vi "InitDrive.vi"   [LabVIEW 2019]
uses:
  <vilib>/Rock Robotics/WPI/ThirdParty/REV Robotics/SPARK MAX/Typedef/Spark MAX Idle Mode.ctl
  refnums.vi
types:
  T1 = typedef "Spark MAX Idle Mode.ctl" = enum16{"Coast", "Brake"}
  T2 = typedef "WPI_MotorControlDeviceRef.ctl" = cluster{"DeviceStatus":errorcluster, "Type":T3, "PWM":cluster{"PWM Channel":T4, "DeadBand":T5}, "CAN":cluster{"Device Number":u8, "SetOutput VI Ref":variant, "GetOutput VI Ref":variant, "Enable VI Ref":variant, "Disable VI Ref":variant, "Data":variant}, "Invert":bool, "DIO PWM":cluster{"PWM \"Enable\" Channel":T4, "DIOChannel":T6, "PWM Rate":dbl}}
  T3 = typedef "WPI_MotorControlType.ctl" = enum16{"PWM", "CAN", "DIO PWM"}
  T4 = typedef "FPGA_DIOPWMChannel.ctl" = enum8{"PWM 0", "PWM 1", "PWM 2", "PWM 3", "PWM 4", "PWM 5", "PWM 6", "PWM 7", "PWM 8", "PWM 9", "PWM MXP 0", "PWM MXP 1", "PWM MXP 2", "PWM MXP 3", "PWM MXP 4", "PWM MXP 5", "PWM MXP 6", "PWM MXP 7", "PWM MXP 8", "PWM MXP 9", "Invalid"}
  T5 = typedef "WPI_PWMDeadband.ctl" = cluster{"Name":string, "maxPositivePwm":i32, "minPositivePwm":i32, "centerPwm":i32, "maxNegativePwm":i32, "minNegativePwm":i32, "angularRange":u16}
  T6 = typedef "FPGA_DIOChannel.ctl" = enum8{"DIO 0", "DIO 1", "DIO 2", "DIO 3", "DIO 4", "DIO 5", "DIO 6", "DIO 7", "DIO 8", "DIO 9", "DIO MXP 0", "DIO MXP 1", "DIO MXP 2", "DIO MXP 3", "DIO MXP 4", "DIO MXP 5", "DIO MXP 6", "DIO MXP 7", "DIO MXP 8", "DIO MXP 9", "DIO MXP 10", "DIO MXP 11", "DIO MXP 12", "DIO MXP 13", "DIO MXP 14", "DIO MXP 15", "SPI Port CS1", "SPI Port CS2", "SPI Port CS3", "SPI Port MISO", "SPI Port MOSI", "Invalid"}
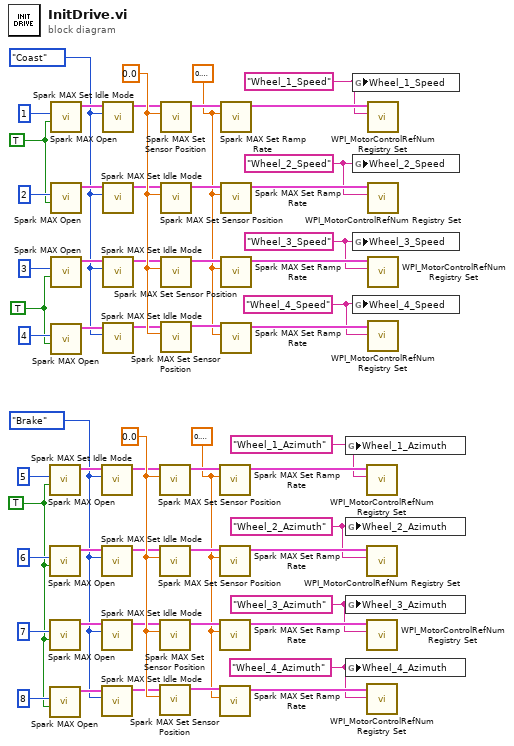
[diagram p0: block diagram]
diagram:
  w1 = TRUE
  w29 = 0.0
  w3 = TRUE
  w5 = "Wheel_3_Azimuth" ("refnum name")
  w4 = "Wheel_4_Azimuth" ("refnum name")
  w6 = "Wheel_2_Azimuth" ("refnum name")
  w2 = Spark_MAX_Idle_Mode."Brake" ("Idle Mode")
  w7 = "Wheel_1_Azimuth" ("refnum name")
  w8 = sgl 0.1 ("Seconds from neutral to full (0)")
  w57 = 0.0
  w31 = TRUE
  w33 = "Wheel_3_Speed" ("refnum name")
  w32 = "Wheel_4_Speed" ("refnum name")
  w34 = "Wheel_2_Speed" ("refnum name")
  w30 = Spark_MAX_Idle_Mode."Coast" ("Idle Mode")
  w35 = "Wheel_1_Speed" ("refnum name")
  w36 = sgl 0.2 ("Seconds from neutral to full (0)")
  n1 = call <vilib>:"Spark MAX Open.vi"("Invert"=w3, "Device Number"=u8 5 ("Drive 1R")) -> ("MotorControlDeviceRef"=w9:T2)  [unwired: 8 in, 1 out]
  n2 = call <vilib>:"Spark MAX Open.vi"("Invert"=w3, "Device Number"=u8 6 ("Drive 2R")) -> ("MotorControlDeviceRef"=w12:T2)  [unwired: 8 in, 1 out]
  n3 = call <vilib>:"Spark MAX Open.vi"("Invert"=w3, "Device Number"=u8 7 ("Drive  3R")) -> ("MotorControlDeviceRef"=w18:T2)  [unwired: 8 in, 1 out]
  n4 = call <vilib>:"Spark MAX Open.vi"("Invert"=w3, "Device Number"=u8 8 ("Drive 4L")) -> ("MotorControlDeviceRef"=w15:T2)  [unwired: 8 in, 1 out]
  n5 = call <vilib>:"Spark MAX Open.vi"("Invert"=w31, "Device Number"=u8 1 ("Drive 1R")) -> ("MotorControlDeviceRef"=w37:T2)  [unwired: 8 in, 1 out]
  n6 = call <vilib>:"Spark MAX Open.vi"("Invert"=w31, "Device Number"=u8 2 ("Drive 2R")) -> ("MotorControlDeviceRef"=w40:T2)  [unwired: 8 in, 1 out]
  n7 = call <vilib>:"Spark MAX Open.vi"("Invert"=w1, "Device Number"=u8 3 ("Drive  3R")) -> ("MotorControlDeviceRef"=w46:T2)  [unwired: 8 in, 1 out]
  n8 = call <vilib>:"Spark MAX Open.vi"("Invert"=w1, "Device Number"=u8 4 ("Drive 4L")) -> ("MotorControlDeviceRef"=w43:T2)  [unwired: 8 in, 1 out]
  n9 = call <vilib>:"Spark MAX Set Idle Mode.vi"("Idle Mode"=w2, "MotorControlDeviceRef in"=w9) -> ("MotorControlDeviceRef out"=w21:T2)  [unwired: 8 in, 1 out]
  n10 = call <vilib>:"Spark MAX Set Idle Mode.vi"("Idle Mode"=w2, "MotorControlDeviceRef in"=w12) -> ("MotorControlDeviceRef out"=w23:T2)  [unwired: 8 in, 1 out]
  n11 = call <vilib>:"Spark MAX Set Idle Mode.vi"("Idle Mode"=w2, "MotorControlDeviceRef in"=w18) -> ("MotorControlDeviceRef out"=w25:T2)  [unwired: 8 in, 1 out]
  n12 = call <vilib>:"Spark MAX Set Idle Mode.vi"("Idle Mode"=w2, "MotorControlDeviceRef in"=w15) -> ("MotorControlDeviceRef out"=w27:T2)  [unwired: 8 in, 1 out]
  n13 = call <vilib>:"Spark MAX Set Idle Mode.vi"("Idle Mode"=w30, "MotorControlDeviceRef in"=w37) -> ("MotorControlDeviceRef out"=w49:T2)  [unwired: 8 in, 1 out]
  n14 = call <vilib>:"Spark MAX Set Idle Mode.vi"("Idle Mode"=w30, "MotorControlDeviceRef in"=w40) -> ("MotorControlDeviceRef out"=w51:T2)  [unwired: 8 in, 1 out]
  n15 = call <vilib>:"Spark MAX Set Idle Mode.vi"("Idle Mode"=w30, "MotorControlDeviceRef in"=w46) -> ("MotorControlDeviceRef out"=w53:T2)  [unwired: 8 in, 1 out]
  n16 = call <vilib>:"Spark MAX Set Idle Mode.vi"("Idle Mode"=w30, "MotorControlDeviceRef in"=w43) -> ("MotorControlDeviceRef out"=w55:T2)  [unwired: 8 in, 1 out]
  n17 = call <vilib>:"Spark MAX Set Sensor Position.vi"("Position"=w29, "MotorControlDeviceRef"=w21) -> ("MotorControlDeviceRef"=w22:T2)  [unwired: 8 in, 1 out]
  n18 = call <vilib>:"Spark MAX Set Sensor Position.vi"("Position"=w29, "MotorControlDeviceRef"=w23) -> ("MotorControlDeviceRef"=w24:T2)  [unwired: 8 in, 1 out]
  n19 = call <vilib>:"Spark MAX Set Sensor Position.vi"("Position"=w29, "MotorControlDeviceRef"=w25) -> ("MotorControlDeviceRef"=w26:T2)  [unwired: 8 in, 1 out]
  n20 = call <vilib>:"Spark MAX Set Sensor Position.vi"("Position"=w29, "MotorControlDeviceRef"=w27) -> ("MotorControlDeviceRef"=w28:T2)  [unwired: 8 in, 1 out]
  n21 = call <vilib>:"Spark MAX Set Sensor Position.vi"("Position"=w57, "MotorControlDeviceRef"=w49) -> ("MotorControlDeviceRef"=w50:T2)  [unwired: 8 in, 1 out]
  n22 = call <vilib>:"Spark MAX Set Sensor Position.vi"("Position"=w57, "MotorControlDeviceRef"=w51) -> ("MotorControlDeviceRef"=w52:T2)  [unwired: 8 in, 1 out]
  n23 = call <vilib>:"Spark MAX Set Sensor Position.vi"("Position"=w57, "MotorControlDeviceRef"=w53) -> ("MotorControlDeviceRef"=w54:T2)  [unwired: 8 in, 1 out]
  n24 = call <vilib>:"Spark MAX Set Sensor Position.vi"("Position"=w57, "MotorControlDeviceRef"=w55) -> ("MotorControlDeviceRef"=w56:T2)  [unwired: 8 in, 1 out]
  n25 = call <vilib>:"Spark MAX Set Ramp Rate.vi"("Seconds from neutral to full (0)"=w8, "MotorControlDeviceRef in"=w22) -> ("MotorControlDeviceRef"=w10:T2)  [unwired: 8 in, 1 out]
  n26 = call <vilib>:"Spark MAX Set Ramp Rate.vi"("Seconds from neutral to full (0)"=w8, "MotorControlDeviceRef in"=w24) -> ("MotorControlDeviceRef"=w14:T2)  [unwired: 8 in, 1 out]
  n27 = call <vilib>:"Spark MAX Set Ramp Rate.vi"("Seconds from neutral to full (0)"=w8, "MotorControlDeviceRef in"=w26) -> ("MotorControlDeviceRef"=w20:T2)  [unwired: 8 in, 1 out]
  n28 = call <vilib>:"Spark MAX Set Ramp Rate.vi"("Seconds from neutral to full (0)"=w8, "MotorControlDeviceRef in"=w28) -> ("MotorControlDeviceRef"=w17:T2)  [unwired: 8 in, 1 out]
  n29 = call <vilib>:"Spark MAX Set Ramp Rate.vi"("Seconds from neutral to full (0)"=w36, "MotorControlDeviceRef in"=w50) -> ("MotorControlDeviceRef"=w38:T2)  [unwired: 8 in, 1 out]
  n30 = call <vilib>:"Spark MAX Set Ramp Rate.vi"("Seconds from neutral to full (0)"=w36, "MotorControlDeviceRef in"=w52) -> ("MotorControlDeviceRef"=w42:T2)  [unwired: 8 in, 1 out]
  n31 = call <vilib>:"Spark MAX Set Ramp Rate.vi"("Seconds from neutral to full (0)"=w36, "MotorControlDeviceRef in"=w54) -> ("MotorControlDeviceRef"=w48:T2)  [unwired: 8 in, 1 out]
  n32 = call <vilib>:"Spark MAX Set Ramp Rate.vi"("Seconds from neutral to full (0)"=w36, "MotorControlDeviceRef in"=w56) -> ("MotorControlDeviceRef"=w45:T2)  [unwired: 8 in, 1 out]
  n33 = global write "refnums.vi" "Wheel_1_Azimuth"(w7) -> ()
  n34 = global write "refnums.vi" "Wheel_2_Azimuth"(w6) -> ()
  n35 = global write "refnums.vi" "Wheel_3_Azimuth"(w5) -> ()
  n36 = global write "refnums.vi" "Wheel_4_Azimuth"(w4) -> ()
  n37 = global write "refnums.vi" "Wheel_1_Speed"(w35) -> ()
  n38 = global write "refnums.vi" "Wheel_2_Speed"(w34) -> ()
  n39 = global write "refnums.vi" "Wheel_3_Speed"(w33) -> ()
  n40 = global write "refnums.vi" "Wheel_4_Speed"(w32) -> ()
  n41 = call <vilib>:"WPI_MotorControlRefNum Registry Set.vi"("refnum name"=w7, "MotorControlDevRef"=w10) -> ()  [unwired: 8 in, 2 out]
  n42 = call <vilib>:"WPI_MotorControlRefNum Registry Set.vi"("refnum name"=w6, "MotorControlDevRef"=w14) -> ()  [unwired: 8 in, 2 out]
  n43 = call <vilib>:"WPI_MotorControlRefNum Registry Set.vi"("refnum name"=w5, "MotorControlDevRef"=w20) -> ()  [unwired: 8 in, 2 out]
  n44 = call <vilib>:"WPI_MotorControlRefNum Registry Set.vi"("refnum name"=w4, "MotorControlDevRef"=w17) -> ()  [unwired: 8 in, 2 out]
  n45 = call <vilib>:"WPI_MotorControlRefNum Registry Set.vi"("refnum name"=w35, "MotorControlDevRef"=w38) -> ()  [unwired: 8 in, 2 out]
  n46 = call <vilib>:"WPI_MotorControlRefNum Registry Set.vi"("refnum name"=w34, "MotorControlDevRef"=w42) -> ()  [unwired: 8 in, 2 out]
  n47 = call <vilib>:"WPI_MotorControlRefNum Registry Set.vi"("refnum name"=w33, "MotorControlDevRef"=w48) -> ()  [unwired: 8 in, 2 out]
  n48 = call <vilib>:"WPI_MotorControlRefNum Registry Set.vi"("refnum name"=w32, "MotorControlDevRef"=w45) -> ()  [unwired: 8 in, 2 out]
